vi "authorize.vi"() -> (3 "Flickr Ref out":refnum<k24>)   [LabVIEW 2012]
uses:
  C:/Users/telsey/Desktop/Personal Projects/Photobooth/Flickr API/FlickrNet-3.5.0/FlickrNet.dll
  FlickrNet-3.5.0/FlickrNet.dll
  <vilib>/Platform/browser.llb/Open URL in Default Browser (string).vi
  <vilib>/LVH/i3 OAuth/i3-oauth.lvlib
panel:
  out "Flickr Ref out 2":refnum<k24>
  in  "User Login Timeout (120000 ms)":i32=120000
  out "remote port":u16
  out "Post Data Transmitted":string
  out "OAuthCalculateAuthorizationUrl":string
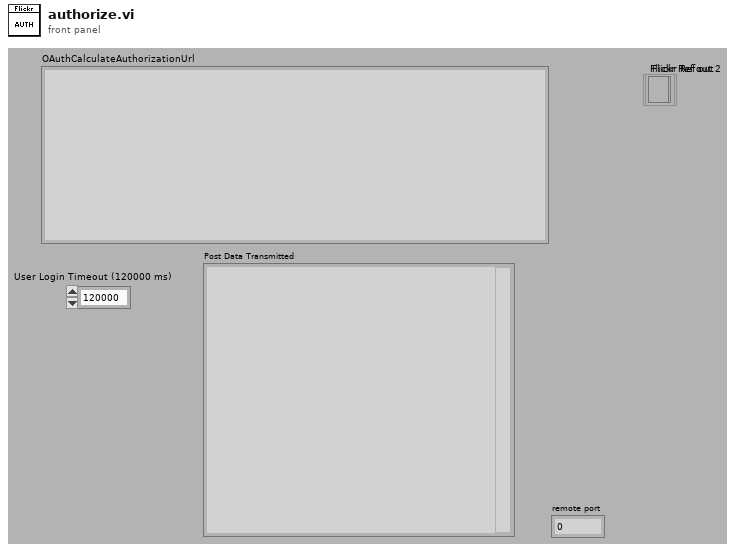
[diagram p1: front panel]
types:
  T1 = enum16{"Standard", "Buffered", "CRLF", "Immediate"}
  T2 = typedef "i3-oauth.lvlib/Name-Value Pair.ctl" = cluster{"Name":string, "Value":string}
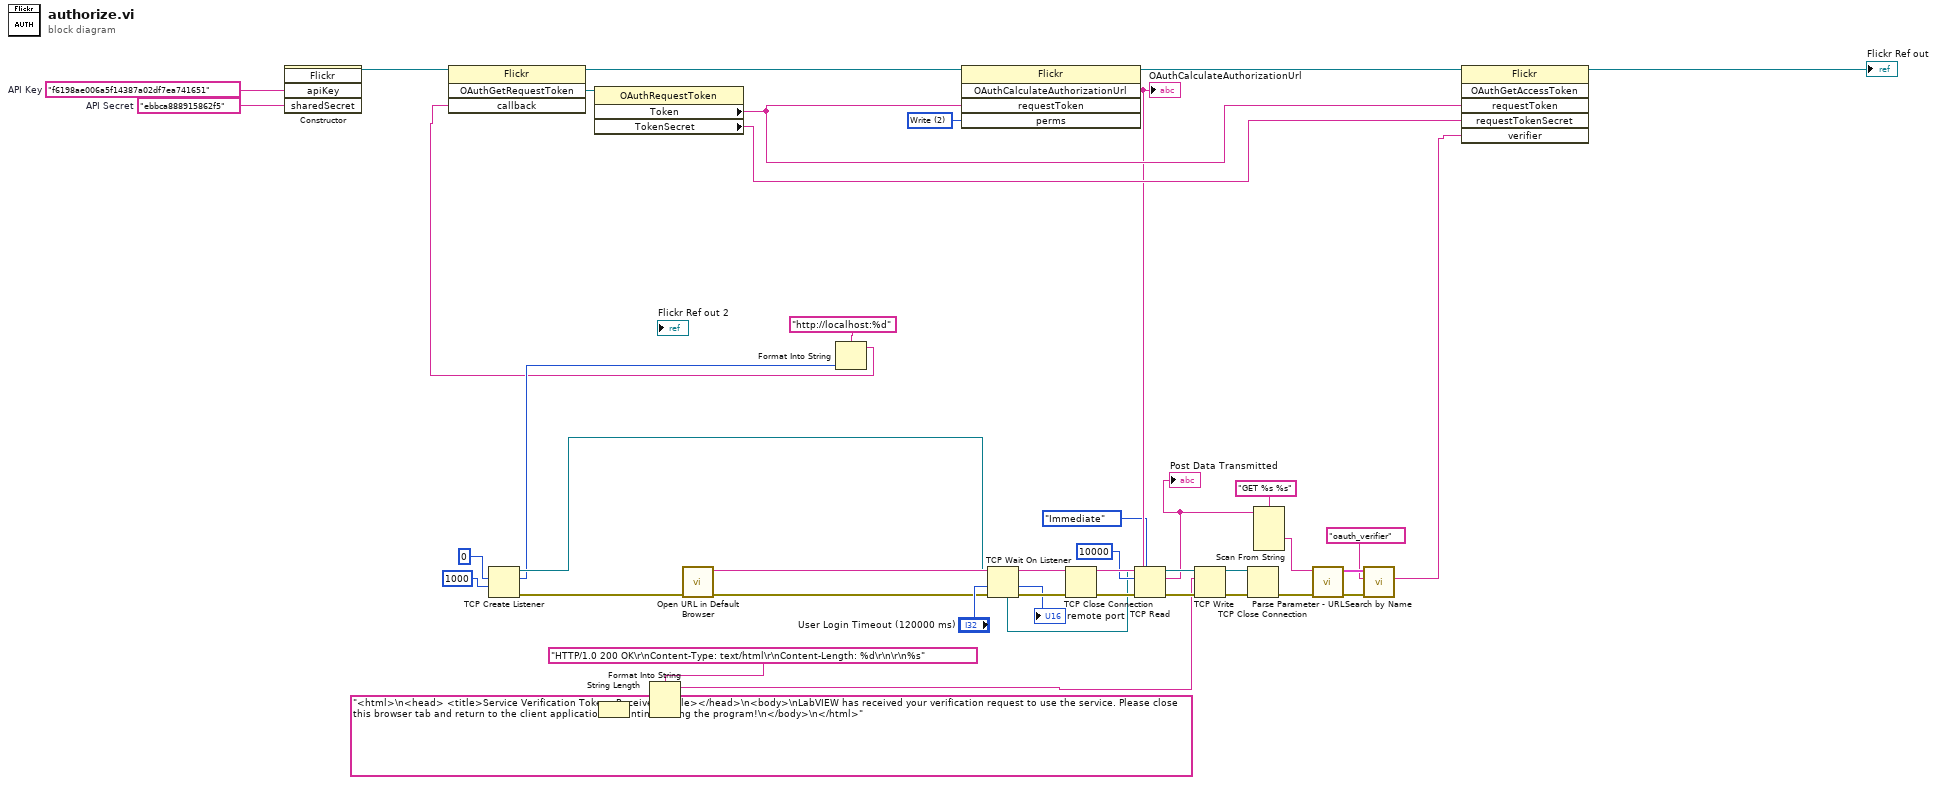
[diagram p0: block diagram]
diagram:
  w2 = "<html>\n<head> <title>Service Verification Tokens Received</title></head>\n<body>\nLabVIEW has received your verification request to use the service. Please close this browser tab and return to the client application to continue using the program!\n</body>\n</html>" ("Callback Response Body")
  w39 = 2 items=["None", "Read", "Write", "Delete"] ("perms")
  w41 = "ebbca888915862f5"  # API Secret
  w42 = "f6198ae006a5f14387a02df7ea741651"  # API Key
  n1 = constructor class="Flickr"("apiKey"=w42, "sharedSecret"=w41) -> (reference out=w40:refnum<k24>)  [unwired: 3 in, 4 out]
  n2 = TCP Create Listener(9:1000 ("timeout ms (25000)"), 10:u16 0 ("port")) -> (0:w12:errorcluster, 2:w7:u16, 3:w19:refnum<k5>)  [unwired: 3 in]
  n3 = String Length(string=w2) -> (length=w3:i32)
  n4 = Format Into String(format string="HTTP/1.0 200 OK\r\nContent-Type: text/html\r\nContent-Length: %d\r\n\r\n%s" ("data in"), w3, w2) -> (resulting string=w1:string)  [unwired: 2 in, 1 out]
  n5 = Format Into String(format string="http://localhost:%d" ("string"), w7) -> (resulting string=w6:string)  [unwired: 2 in, 1 out]
  n6 = invoke class="Flickr" method="OAuthGetRequestToken"(reference=w40, "callback"=w6) -> (reference out=w36:refnum<k24>, "OAuthGetRequestToken"=w35:refnum<k24>)  [unwired: 2 in, 2 out]
  n7 = property class="OAuthRequestToken"(reference=w35) -> ("Token"=w34:string, "TokenSecret"=w37:string)  [unwired: 1 in, 2 out]
  n8 = invoke class="Flickr" method="OAuthCalculateAuthorizationUrl"(reference=w36, "requestToken"=w34, "perms"=w39) -> (reference out=w38:refnum<k24>, "OAuthCalculateAuthorizationUrl"=w33:string)  [unwired: 2 in, 3 out]
  "OAuthCalculateAuthorizationUrl" <- w33
  n9 = call-poly <vilib>:"Open URL in Default Browser.vi"("error in (no error)"=w12, "URL"=w33) -> ("error out"=w11:errorcluster)  [unwired: 4 in, 1 out]
  n10 = TCP Wait On Listener(8:w11, 9:"User Login Timeout (120000 ms)", 11:w19) -> (0:w17:errorcluster, 1:→"remote port":u16, 3:w15:refnum<k5>, 4:w14:refnum<k5>)  [unwired: 1 in, 1 out]
  n11 = TCP Close Connection(connection ID=w15, error in (no error)=w17) -> (error out=w16:errorcluster)  [unwired: 1 in, 1 out]
  n12 = TCP Read(connection ID=w14, bytes to read=10000, error in (no error)=w16, 7:T1."Immediate" ("mode (standard)")) -> (connection ID out=w31:refnum<k5>, data out=w9:string, error out=w30:errorcluster)  [unwired: 1 in]
  "Post Data Transmitted" <- w9
  n13 = TCP Write(connection ID=w31, data in=w1, error in (no error)=w30) -> (connection ID out=w28:refnum<k5>, error out=w29:errorcluster)  [unwired: 1 in, 1 out]
  n14 = TCP Close Connection(connection ID=w28, error in (no error)=w29) -> (error out=w26:errorcluster)  [unwired: 1 in, 1 out]
  n15 = Scan From String(format string="GET %s %s", input string=w9) -> (output 1=w23:string)  [unwired: 5 in, 3 out]
  n16 = call <vilib>:"Parse Parameter - URL.vi"("error in (no error)"=w26, "URL"=w23) -> ("error out"=w25:errorcluster, "URL Parameters"=w22:T2[])  [unwired: 8 in]
  n17 = call <vilib>:"Search by Name.vi"("error in (no error)"=w25, "Name"="oauth_verifier" ("Key"), "Name-Value Pair List"=w22) -> ("Value"=w5:string)  [unwired: 6 in, 2 out]
  n18 = invoke class="Flickr" method="OAuthGetAccessToken"(reference=w38, "requestToken"=w34, "requestTokenSecret"=w37, "verifier"=w5) -> (reference out=→"Flickr Ref out":refnum<k24>)  [unwired: 2 in, 5 out]
